vi "WPI_SerialPortTermination.vi"(8 "error in (no error)":errorcluster, 9 "Termination Char (0xA = '\\n' = LF)":u8=10 format="%.0x", 10 "Enable? (T)":bool=TRUE, 11 "SerialPortRef":T1) -> (0 "error out":errorcluster, 3 "SerialPortRef":T1)   [LabVIEW 2017]
doc: "Specifies whether to terminate a read operation with a termination character.\n\nThis software is licensed. Open the labview\\readme\\WPI Robotics Library Open Source License.txt file for more information."
uses:
  <vilib>/Rock Robotics/WPI/SerialPort/WPI_SerialPortRef.ctl
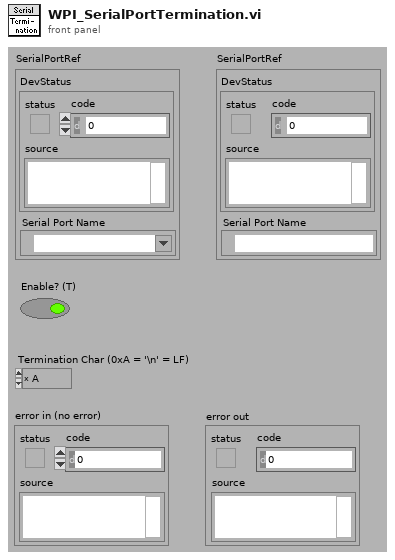
[diagram p1: front panel]
types:
  T1 = typedef "WPI_SerialPortRef.ctl" = cluster{"DevStatus":errorcluster, "Serial Port Name":refnum<visa-resource-name>}
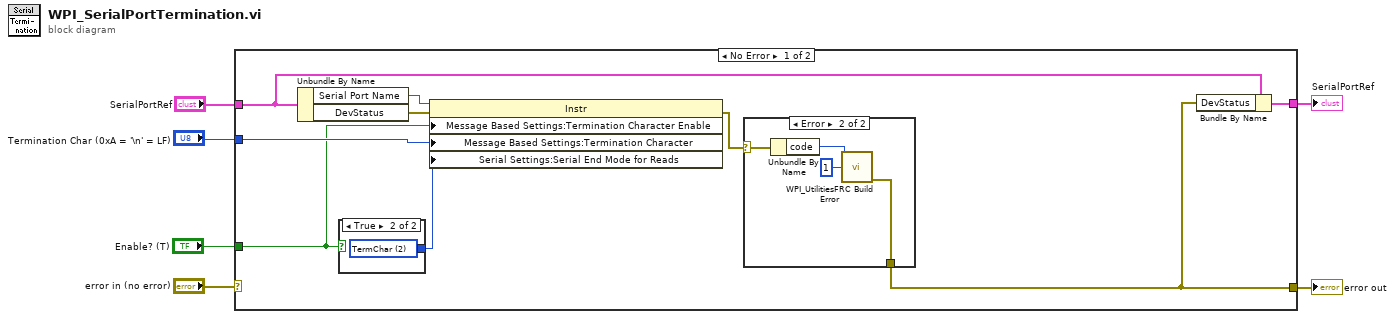
[diagram p0: block diagram]
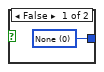
[diagram p2: hidden frame]
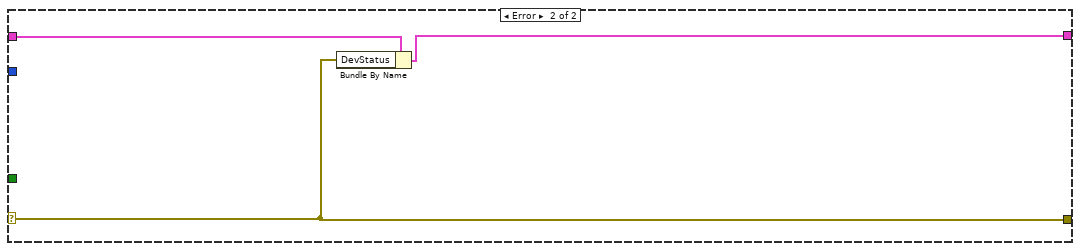
[diagram p4: hidden frame]
diagram:
  n1 = case shown="No Error" "error in (no error)" {
    selector: "error in (no error)" -> [_ w23]
    tunnel: "SerialPortRef" -> [w12 w25]
    tunnel: "Termination Char (0xA = '\\n' = LF)" -> [w15 _]
    tunnel: [w11 w24] -> w4
    tunnel: [w7 w23] -> w2
    tunnel: "Enable? (T)" -> [w9 _]
    frame No Error {
      n2 = Unbundle By Name(w12) -> ("Serial Port Name"=w14:refnum<visa-resource-name>, "DevStatus"=w13:errorcluster)
      n3 = case shown="True" w9 {
        tunnel: [w16 w17] -> w10
        frame False {
          w16 = u16 0 items=["None", "LastBit", "TermChar"] ("Serial Settings:Serial End Mode for Reads")
        }
        frame True {
          w17 = u16 2 items=["None", "LastBit", "TermChar"] ("Serial Settings:Serial End Mode for Reads")
        }
      }
      n4 = property class="Instr"(reference=w14, error in=w13, "Message Based Settings:Termination Character Enable"=w9, "Message Based Settings:Termination Character"=w15, "Serial Settings:Serial End Mode for Reads"=w10) -> (error out=w8:errorcluster)  [unwired: 1 in]
      n5 = case shown="Error" w8 {
        selector: w8 -> [w18 w20]
        tunnel: [w18 w19] -> w7
        frame No Error {
        }
        frame Error {
          n6 = Unbundle By Name(w20) -> ("code"=w22:i32)
          n7 = call <vilib>:"WPI_UtilitiesFRC Build Error.vi"("error code"=w22, "chain levels to remove (1)"=1) -> ("error out"=w19:errorcluster)  [unwired: 3 in, 10 out]
        }
      }
      n8 = Bundle By Name(cluster=w12, "DevStatus"=w7) -> (w11:T1)
    }
    frame Error {
      n9 = Bundle By Name(cluster=w25, "DevStatus"=w23) -> (w24:T1)
    }
  }
  "error out" <- w2
  "SerialPortRef" <- w4
